vi "Read State.vi"(8 "error in (no error)":errorcluster, 10 "Trigger":bool, 11 "SciShutt in":refnum<class "SciShutt.lvclass">) -> (0 "error out":errorcluster, 2 "Set":T1, 3 "SciShutt out":refnum<class "SciShutt.lvclass">)   [LabVIEW 2016, in "SciShutt.lvclass"]
uses:
  SciShutt.lvclass
  Controls/Shutter States.ctl
  BiStable/BiStableShutter.lvclass
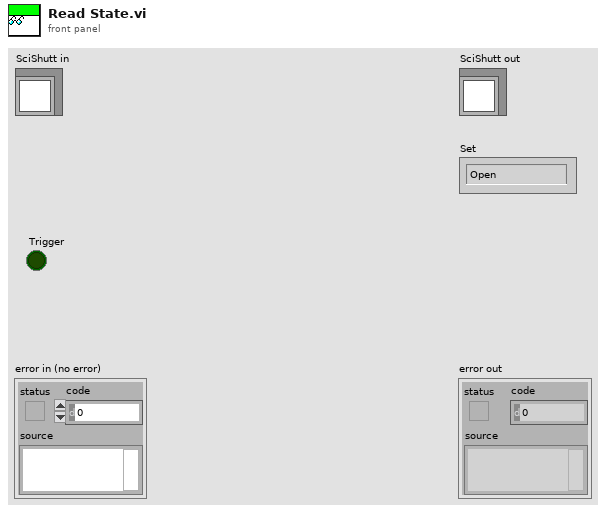
[diagram p1: front panel]
types:
  T1 = typedef "Shutter States.ctl" = enum16{"Open", "Close", "Wait", "Off", "Arm", "Idle"}
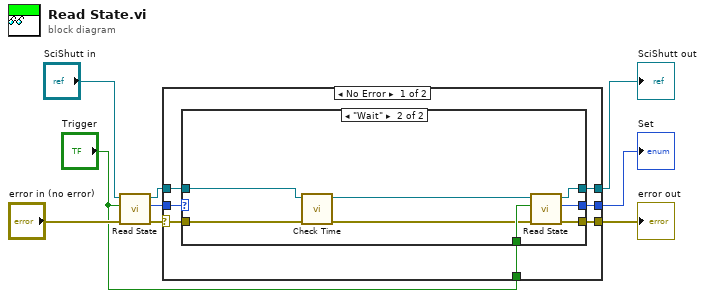
[diagram p0: block diagram]
diagram:
  n1 = call-parent "Read State.vi"("error in (no error)"="error in (no error)", "Trigger"="Trigger", "Shutter in"="SciShutt in") -> ("error out"=w7:errorcluster, "Set"=w3:T1, "Shutter out"=w6:refnum<class "SciShutt.lvclass">)  [unwired: 6 in]
  n2 = case shown="No Error" w7 {
    selector: w7 -> [w15 w28]
    tunnel: w6 -> [w16 w30]
    tunnel: [w11 w29] -> w5
    tunnel: [w13 w30] -> w1
    tunnel: [w14 w28] -> w4
    tunnel: w3 -> [w12 w29]
    tunnel: "Trigger" -> [w10 _]
    frame No Error {
      n3 = case shown="\"Wait\"" w12 {
        selector: w12 -> [w19 _]
        tunnel: w16 -> [w18 w27]
        tunnel: w15 -> [w17 w26]
        tunnel: [w17 w22] -> w14
        tunnel: [w18 w24] -> w13
        tunnel: [w19 w23] -> w11
        tunnel: w10 -> [_ w21]
        frame Default {
        }
        frame "Wait" {
          n4 = call-dynamic "Check Time.vi"("error in (no error)"=w26, "BiStableShutter in"=w27) -> ("error out"=w20:errorcluster, "BiStableShutter out"=w25:refnum<class "SciShutt.lvclass">)  [unwired: 8 in]
          n5 = call-parent "Read State.vi"("error in (no error)"=w20, "Trigger"=w21, "Shutter in"=w25) -> ("error out"=w22:errorcluster, "Set"=w23:T1, "Shutter out"=w24:refnum<class "SciShutt.lvclass">)  [unwired: 6 in]
        }
      }
    }
    frame Error {
    }
  }
  "error out" <- w4
  "SciShutt out" <- w1
  "Set" <- w5
